vi "Test JeVois Read.vi"() -> ()   [LabVIEW 2017]
panel:
  out "concatenated string":string
  in  "stop":bool
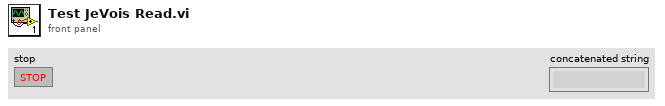
[diagram p1: front panel]
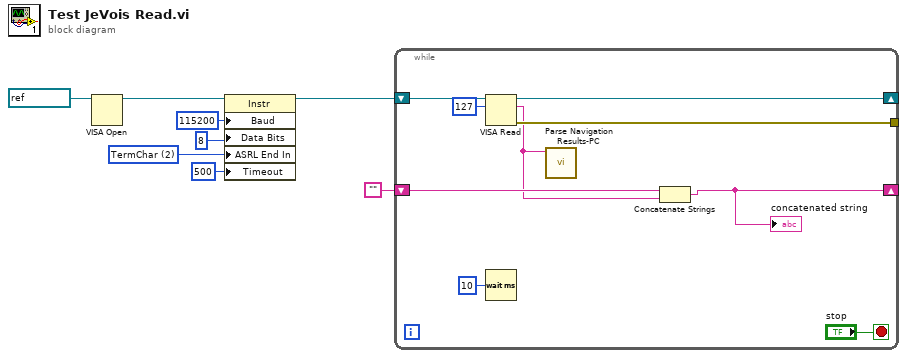
[diagram p0: block diagram]
diagram:
  w4 = u16 2 items=["None", "Last Bit", "TermChar"] ("Serial Settings:End Mode for Reads")
  n1 = VISA Open(VISA resource name=refnum<visa-resource-name> "COM2") -> (VISA resource name=w7:refnum<visa-resource-name>)  [unwired: 4 in, 1 out]
  n2 = property class="Instr"(reference=w7, "Baud"=u32 115200 ("Serial Settings:Baud Rate"), "Data Bits"=u16 8 ("Serial Settings:Data Bits"), "ASRL End In"=w4, "Timeout"=u32 500 ("General Settings:Timeout Value")) -> (reference out=w3:refnum<visa-resource-name>)  [unwired: 1 in, 1 out]
  n3 = while {
    shift-right: [w13] -> _
    shift-left: w3 -> [w15]
    tunnel: [w12] -> _
    shift-right: [w9] -> _
    shift-left: "" -> [w11]
    stop <- "stop" stop-if-true
    n4 = VISA Read(VISA resource name=w15, byte count=u32 127) -> (VISA resource name out=w13:refnum<visa-resource-name>, read buffer=w10:string, error out=w12:errorcluster)  [unwired: 1 in, 1 out]
    n5 = Wait (ms)(milliseconds to wait=u32 10) -> ()  [unwired: 1 out]
    n6 = call "Parse Navigation Results-PC.vi"("String"=w10) -> ()  [unwired: 11 in]
    n7 = Concatenate Strings(w11, w10) -> (w9:string)
    "concatenated string" <- w9
  }
